vi "Scale array.vi"(2 "有边缘？":bool=TRUE, 3 "Scale":u8=1 min=1, 5 "in Array":bool[][](array[boolean])=[[TRUE, TRUE, TRUE, TRUE, TRUE, TRUE, TRUE, FALSE, FALSE, TRUE, TRUE, FALSE, FALSE, FALSE, TRUE, TRUE, TRUE, TRUE, TRUE, TRUE, TRUE], [TRUE, FALSE, FALSE, FALSE, FALSE, FALSE, TRUE, FALSE, FALSE, TRUE, FALSE, TRUE, FALSE, FALSE, TRUE, FALSE, FALSE, FALSE, FALSE, FALSE, TRUE], [TRUE, FALSE, TRUE, TRUE, TRUE, FALSE, TRUE, FALSE, FALSE, TRUE, FALSE, TRUE, TRUE, FALSE, TRUE, FALSE, TRUE, TRUE, TRUE, FALSE, TRUE], [TRUE, FALSE, TRUE, TRUE, TRUE, FALSE, TRUE, FALSE, TRUE, TRUE, TRUE, TRUE, TRUE, FALSE, TRUE, FALSE, TRUE, TRUE, TRUE, FALSE, TRUE], [TRUE, FALSE, TRUE, TRUE, TRUE, FALSE, TRUE, FALSE, TRUE, TRUE, TRUE, FALSE, TRUE, FALSE, TRUE, FALSE, TRUE, TRUE, TRUE, FALSE, TRUE], [TRUE, FALSE, FALSE, FALSE, FALSE, FALSE, TRUE, FALSE, FALSE, TRUE, FALSE, FALSE, FALSE, FALSE, TRUE, FALSE, FALSE, FALSE, FALSE, FALSE, TRUE], [TRUE, TRUE, TRUE, TRUE, TRUE, TRUE, TRUE, FALSE, TRUE, FALSE, TRUE, FALSE, TRUE, FALSE, TRUE, TRUE, TRUE, TRUE, TRUE, TRUE, TRUE], [FALSE, FALSE, FALSE, FALSE, FALSE, FALSE, FALSE, FALSE, TRUE, FALSE, FALSE, TRUE, FALSE, FALSE, FALSE, FALSE, FALSE, FALSE, FALSE, FALSE, FALSE], [FALSE, FALSE, TRUE, TRUE, FALSE, FALSE, TRUE, FALSE, FALSE, FALSE, FALSE, TRUE, TRUE, TRUE, TRUE, FALSE, TRUE, TRUE, FALSE, FALSE, FALSE], [TRUE, FALSE, FALSE, TRUE, TRUE, FALSE, FALSE, FALSE, TRUE, FALSE, TRUE, FALSE, FALSE, FALSE, TRUE, FALSE, TRUE, FALSE, TRUE, TRUE, FALSE], [FALSE, FALSE, TRUE, FALSE, FALSE, TRUE, TRUE, TRUE, TRUE, TRUE, FALSE, FALSE, FALSE, TRUE, FALSE, FALSE, FALSE, TRUE, FALSE, FALSE, TRUE], [FALSE, TRUE, TRUE, TRUE, TRUE, FALSE, FALSE, TRUE, TRUE, FALSE, TRUE, FALSE, TRUE, TRUE, TRUE, TRUE, FALSE, FALSE, TRUE, FALSE, TRUE], [TRUE, TRUE, TRUE, FALSE, FALSE, TRUE, TRUE, FALSE, FALSE, FALSE, TRUE, TRUE, FALSE, TRUE, TRUE, FALSE, FALSE, FALSE, TRUE, FALSE, TRUE], [FALSE, FALSE, FALSE, FALSE, FALSE, FALSE, FALSE, FALSE, FALSE, FALSE, FALSE, TRUE, FALSE, FALSE, FALSE, TRUE, TRUE, FALSE, TRUE, FALSE, TRUE], [TRUE, TRUE, TRUE, TRUE, TRUE, TRUE, TRUE, FALSE, FALSE, TRUE, FALSE, TRUE, TRUE, TRUE, FALSE, FALSE, TRUE, FALSE, FALSE, TRUE, FALSE], [TRUE, FALSE, FALSE, FALSE, FALSE, FALSE, TRUE, FALSE, FALSE, TRUE, TRUE, TRUE, TRUE, FALSE, FALSE, FALSE, FALSE, FALSE, TRUE, FALSE, TRUE], [TRUE, FALSE, TRUE, TRUE, TRUE, FALSE, TRUE, FALSE, FALSE, TRUE, FALSE, TRUE, TRUE, FALSE, FALSE, FALSE, TRUE, TRUE, TRUE, TRUE, FALSE], [TRUE, FALSE, TRUE, TRUE, TRUE, FALSE, TRUE, FALSE, TRUE, TRUE, TRUE, TRUE, FALSE, TRUE, FALSE, TRUE, TRUE, FALSE, TRUE, TRUE, FALSE], [TRUE, FALSE, TRUE, TRUE, TRUE, FALSE, TRUE, FALSE, TRUE, TRUE, FALSE, TRUE, TRUE, TRUE, FALSE, FALSE, TRUE, TRUE, FALSE, FALSE, TRUE], [TRUE, FALSE, FALSE, FALSE, FALSE, FALSE, TRUE, FALSE, FALSE, FALSE, FALSE, FALSE, TRUE, FALSE, TRUE, TRUE, FALSE, FALSE, TRUE, TRUE, TRUE], [TRUE, TRUE, TRUE, TRUE, TRUE, TRUE, TRUE, FALSE, FALSE, TRUE, TRUE, TRUE, TRUE, FALSE, TRUE, FALSE, TRUE, FALSE, TRUE, FALSE, FALSE]]) -> (0 "out Array":bool[][](array[boolean]), 1 "大小":i32[](array[numeric]))   [LabVIEW 2018]
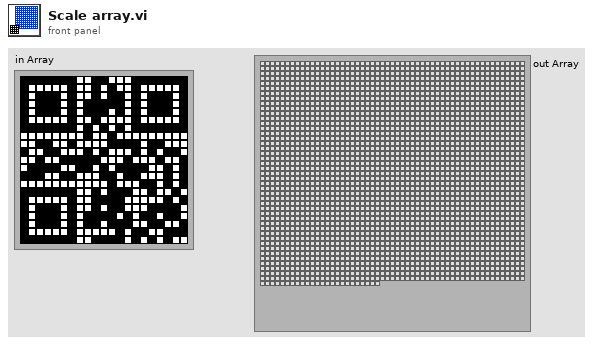
[diagram p1: front panel]
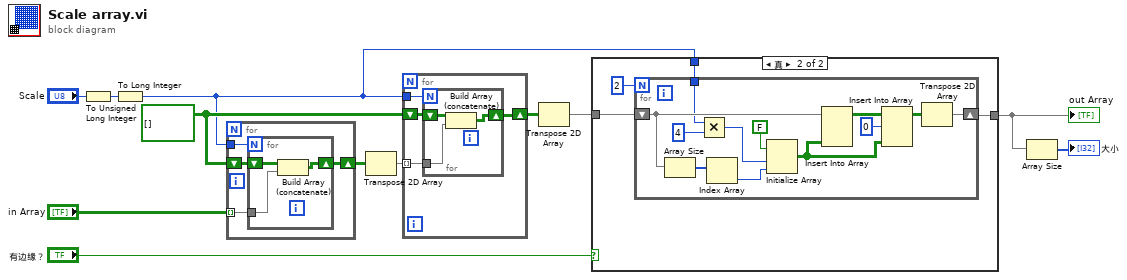
[diagram p0: block diagram]
diagram:
  w11 = bool[][] [] ("out Array")
  n1 = To Unsigned Long Integer(number="Scale") -> (unsigned 32bit integer=w6:u32)
  n2 = To Long Integer(number=w6) -> (32bit integer=w1:i32)
  n3 = for {
    tunnel: "in Array" -> [w14] mode=indexing
    shift-right: [w13] -> w10
    shift-left: w11 -> [w16]
    tunnel: w1 -> [w15]
    n4 = for {
      N: w15 -> [_]
      tunnel: w14 -> [w17]
      shift-right: [w18] -> w13
      shift-left: w16 -> [w19]
      n5 = Build Array (concatenate)(w19, w17) -> (w18:bool[][])
    }
  }
  n6 = Transpose 2D Array(2D array=w10) -> (transposed array=w9:bool[][])
  n7 = for {
    tunnel: w9 -> [w23] mode=indexing
    tunnel: w1 -> [w22]
    shift-right: [w20] -> w8
    shift-left: w11 -> [w21]
    n8 = for {
      N: w22 -> [_]
      tunnel: w23 -> [w25]
      shift-right: [w24] -> w20
      shift-left: w21 -> [w26]
      n9 = Build Array (concatenate)(w26, w25) -> (w24:bool[][])
    }
  }
  n10 = Transpose 2D Array(2D array=w8) -> (transposed array=w5:bool[][])
  n11 = case shown="真" "有边缘？" {
    tunnel: w5 -> [w27 w31]
    tunnel: [w27 w29] -> w3
    tunnel: w1 -> [_ w28]
    frame False {
    }
    frame True {
      n12 = for {
        N: 2 -> [_]
        shift-right: [w35] -> w29
        shift-left: w31 -> [w40]
        tunnel: w28 -> [w32]
        n13 = Array Size(array=w40) -> (size(s)=w43:i32[])
        n14 = Multiply(x=w32, y=4 ("维数大小")) -> (x*y=w34:i32)
        n15 = Index Array(array=w43) -> (element=w41:i32)  [unwired: 1 in]
        n16 = Initialize Array(FALSE, w34, w41) -> (w37:bool[][])
        n17 = Insert Into Array(array=w40, new element=w37) -> (w39:bool[][])  [unwired: 2 in]
        n18 = Insert Into Array(array=w39, index (row)=0 ("索引 (行)"), new element=w37) -> (w36:bool[][])  [unwired: 1 in]
        n19 = Transpose 2D Array(2D array=w36) -> (transposed array=w35:bool[][])
      }
    }
  }
  "out Array" <- w3
  n20 = Array Size(array=w3) -> (size(s)=→"大小":i32[])
